vi "Create_EIP_waveform_Channel 2.vi"(9 "Mapped":dbl, 10 "time":timestamp, 11 "EIP":dbl) -> (3 "waveform_array":waveform(dbl)[](array[waveform])=[{"t0"=timestamp(0 s since 1904-01-01), "dt"=1.0, "Y"=[]}, {"t0"=timestamp(3732035173.078092 s since 1904-01-01), "dt"=1.0, "Y"=[302.8589782714844], "attributes"=variant("NI_ChannelName"=variant(string "T1"))}])   [LabVIEW 2019]
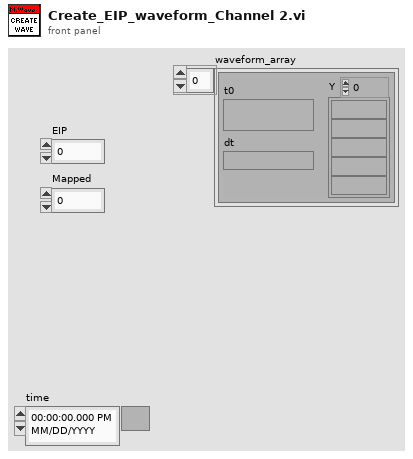
[diagram p1: front panel]
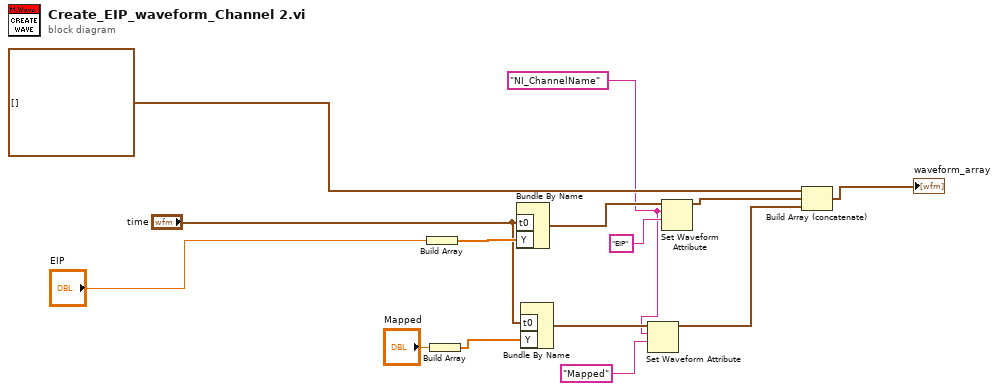
[diagram p0: block diagram]
diagram:
  w1 = "NI_ChannelName" ("name")
  n1 = Build Array("EIP") -> (w12:dbl[])
  n2 = Build Array("Mapped") -> (w6:dbl[])
  n3 = Bundle By Name("t0"="time", "Y"=w12) -> (w8:waveform(dbl))  [unwired: 1 in]
  n4 = Bundle By Name("t0"="time", "Y"=w6) -> (w11:waveform(dbl))  [unwired: 1 in]
  n5 = Set Waveform Attribute(5:"Mapped" ("name"), 6:w1, 7:w11) -> (3:w3:waveform(dbl))  [unwired: 1 in, 2 out]
  n6 = Set Waveform Attribute(5:"EIP" ("name"), 6:w1, 7:w8) -> (3:w7:waveform(dbl))  [unwired: 1 in, 2 out]
  n7 = Build Array (concatenate)(waveform(dbl)[] [], w7, w3) -> (→"waveform_array":waveform(dbl)[])
